vi "GV_YzoomLimit.vi"(6 "Zoom In/Out":bool, 8 "error in (no error)":errorcluster, 11 "Gviewer in":refnum<class "Gviewer.lvclass">) -> (0 "error out":errorcluster, 1 "Allowed":bool, 3 "Gviewer out":refnum<class "Gviewer.lvclass">)   [LabVIEW 2020, in "Sgraph_lib_V1.lvlib" / "Gviewer.lvclass"]
doc: "Determine if Y scrollwheel zoom is still allowed (within limits?)"
uses:
  Gviewer.lvclass
  Gviewer.lvclass/Gviewer.ctl
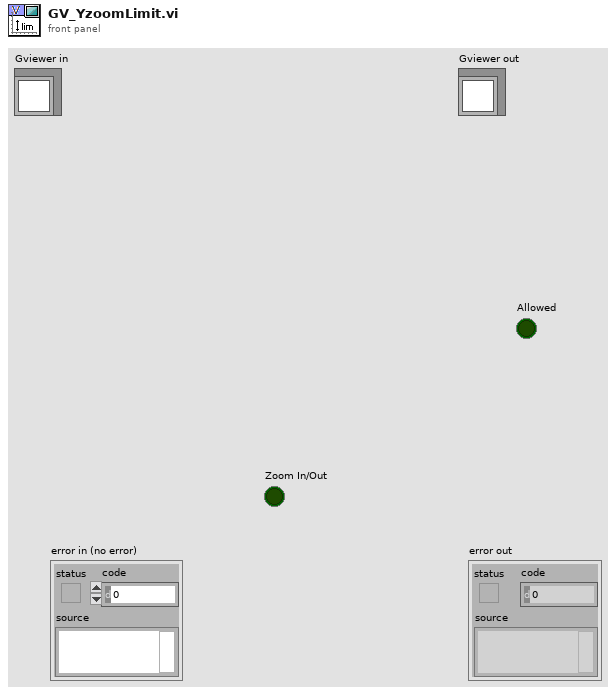
[diagram p1: front panel]
types:
  T1 = typedef "Sgraph_lib_V1.lvlib/Gviewer.lvclass/Typedef_SelProperties.ctl" = cluster{"Color":u32, "LineType":T2, "max":dbl, "min":dbl, "unit":string}
  T2 = typedef "Sgraph_lib_V1.lvlib/Gviewer.lvclass/Typedef_LineType.ctl" = enum16{"num_bare", "num_MinMax_Area", "num_MinMax_Lines", "num_MinMax_Forfor", "num_Max_Area", "num_Max_Line", "num_Max_Forfor", "num_Min_Area", "num_Min_Line", "num_Min_Fosfor", "Boolean_Line_01", "Boolean_Area_01", "Boolean_Fosfor_01", "Boolean_Line_TF", "Boolean_Area_TF", "Boolean_Fosfor_TF", "Boolean_OnOff_Line", "Boolean_OnOff_Area", "Boolean_OnOff_Fosfor", "Boolean_spare", "StringEvent_Line", "StringEvent_TimeLine"}
  T3 = cluster{"data":dbl[], "max":dbl[], "min":dbl[], "Status":u32[]}[]
  T4 = typedef "LVRectTypeDef.ctl" = cluster{"Left":i16, "Top":i16, "Right":i16, "Bottom":i16}
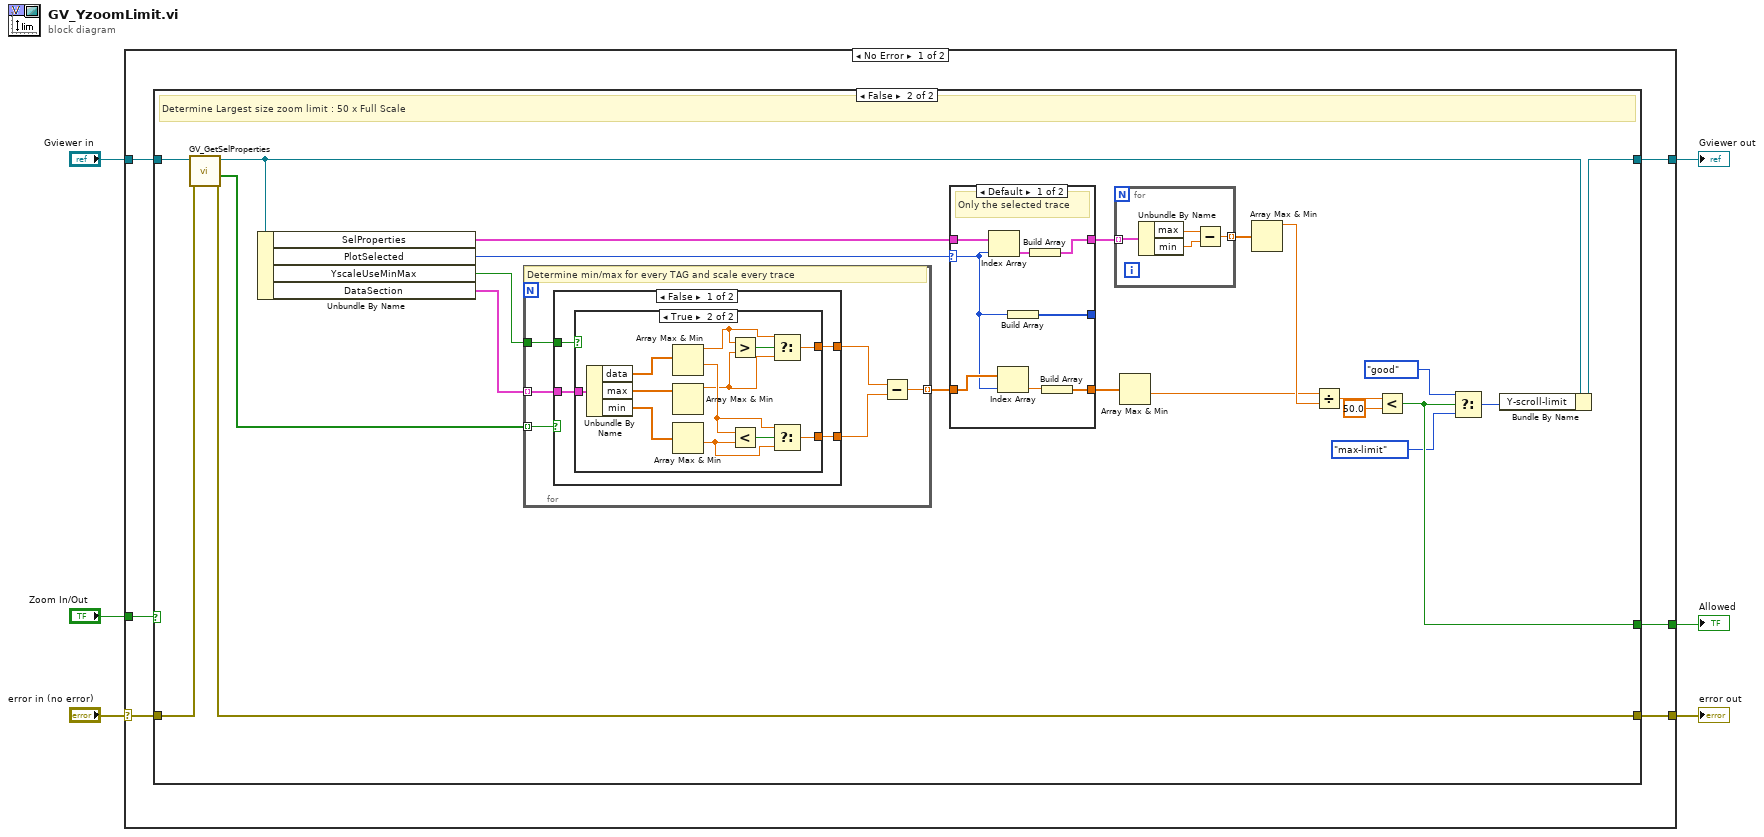
[diagram p0: block diagram]
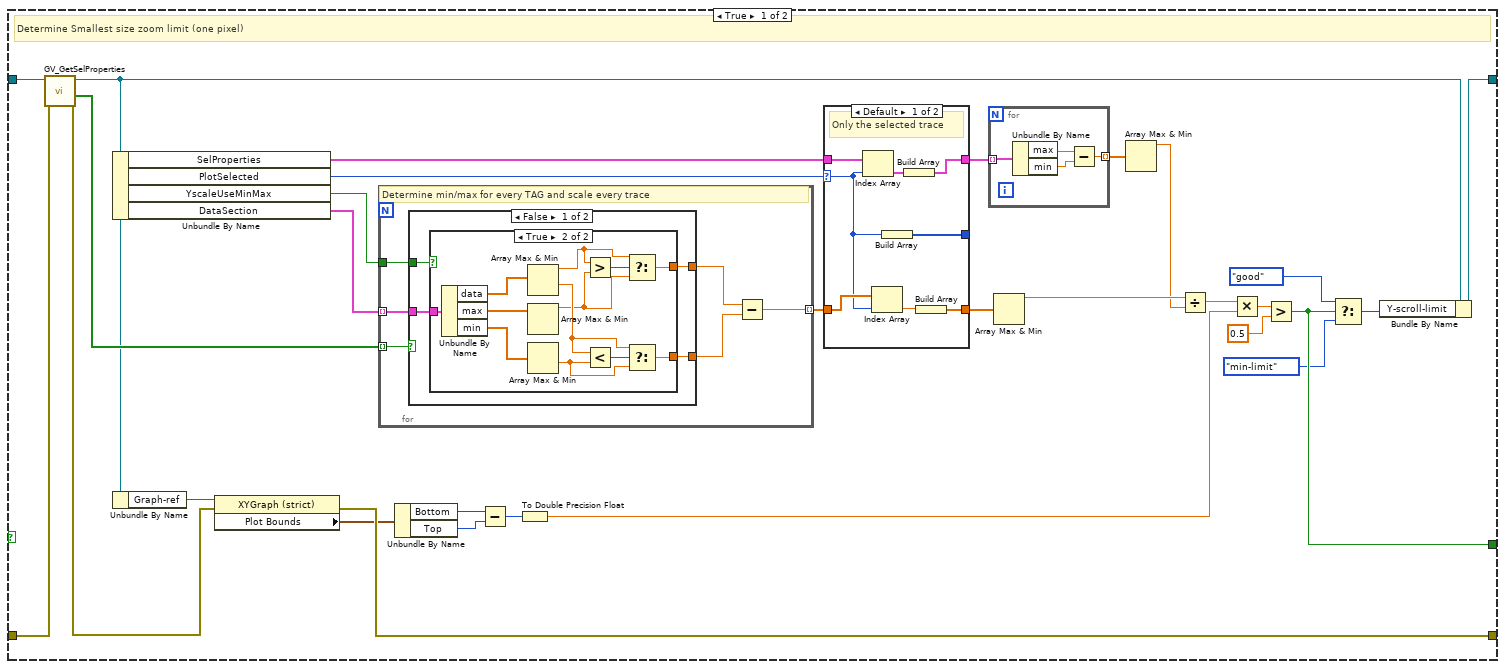
[diagram p2: hidden frame]
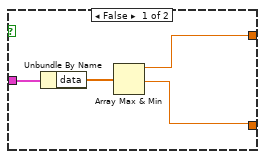
[diagram p3: hidden frame]
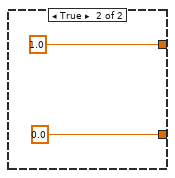
[diagram p4: hidden frame]
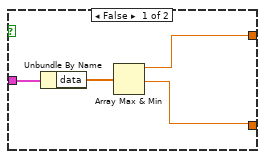
[diagram p6: hidden frame]
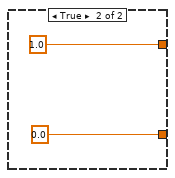
[diagram p7: hidden frame]
diagram:
  n1 = case shown="No Error" "error in (no error)" {
    selector: "error in (no error)" -> [w11 w154]
    tunnel: [w9 w154] -> w5
    tunnel: [w10 w153] -> w3
    tunnel: "Gviewer in" -> [w12 w153]
    tunnel: [w8 _] -> w2
    tunnel: "Zoom In/Out" -> [w7 _]
    frame No Error {
      n2 = case shown="False" w7 {
        tunnel: w12 -> [w40 w106]
        tunnel: w11 -> [w38 w104]
        tunnel: [w15 w87] -> w10
        tunnel: [w31 w97] -> w9
        tunnel: [w17 w92] -> w8
        frame True {
          # "Determine Smallest size zoom limit (one pixel)"
          n3 = call "GV_GetSelProperties.vi"("error in (no error)"=w38, "Gviewer in"=w40) -> ("error out"=w32:errorcluster, "Bool_id"=w39:bool[], "Gviewer out"=w16:refnum<class "Gviewer.lvclass">)  [unwired: 6 in, 1 out]
          n4 = Unbundle By Name(w16) -> ("SelProperties"=w37:T1[], "PlotSelected"=w42:i32, "YscaleUseMinMax"=w41:bool, "DataSection"=w36:T3)
          n5 = Unbundle By Name(w16) -> ("Graph-ref"=w33:refnum<vi>)
          n6 = property class="XYGraph (strict)"(reference=w33, error in=w32) -> (error out=w31:errorcluster, "Plot Bounds"=w30:T4)  [unwired: 1 out]
          n7 = for {
            tunnel: w41 -> [w52]
            tunnel: w36 -> [w51] mode=indexing
            tunnel: w39 -> [w50] mode=indexing
            tunnel: [w47] -> w35 mode=indexing
            # "Determine min/max for every TAG and scale every trace"
            n8 = case shown="False" w50 {
              tunnel: w52 -> [w56 _]
              tunnel: w51 -> [w55 _]
              tunnel: [w54 1.0] -> w49
              tunnel: [w53 0.0] -> w48
              frame False {
                n9 = case shown="True" w56 {
                  tunnel: w55 -> [w59 w72]
                  tunnel: [w58 w64] -> w54
                  tunnel: [w57 w63] -> w53
                  frame False {
                    n10 = Unbundle By Name(w59) -> ("data"=w60:dbl[])
                    n11 = Array Max & Min(array=w60) -> (max value=w58:dbl, min value=w57:dbl)  [unwired: 2 out]
                  }
                  frame True {
                    n12 = Unbundle By Name(w72) -> ("data"=w71:dbl[], "max"=w70:dbl[], "min"=w69:dbl[])
                    n13 = Array Max & Min(array=w71) -> (max value=w62:dbl, min value=w65:dbl)  [unwired: 2 out]
                    n14 = Array Max & Min(array=w70) -> (max value=w61:dbl)  [unwired: 3 out]
                    n15 = Array Max & Min(array=w69) -> (min value=w66:dbl)  [unwired: 3 out]
                    n16 = Greater?(x=w62, y=w61) -> (0:w68:bool)
                    n17 = Less?(x=w65, y=w66) -> (x < y?=w67:bool)
                    n18 = Select(t=w62, s=w68, f=w61) -> (s? t:f=w64:dbl)
                    n19 = Select(t=w65, s=w67, f=w66) -> (s? t:f=w63:dbl)
                  }
                }
              }
              frame True {
              }
            }
            n20 = Subtract(x=w49, y=w48) -> (x-y=w47:dbl)
          }
          n21 = Unbundle By Name(w30) -> ("Bottom"=w29:i16, "Top"=w28:i16)
          n22 = Subtract(x=w29, y=w28) -> (x-y=w24:i16)
          n23 = To Double Precision Float(number=w24) -> (double precision float=w21:dbl)
          n24 = case shown="Default" w42 {
            selector: w42 -> [w77 _]
            tunnel: w37 -> [w81 w83]
            tunnel: [w82 w83] -> w27
            tunnel: [w79 w85] -> _
            tunnel: w35 -> [w78 w84]
            tunnel: [w75 w84] -> w34
            frame Default {
              # "Only the selected trace"
              n25 = Index Array(array=w81, index=w77) -> (element=w80:T1)
              n26 = Index Array(array=w78, index=w77) -> (element=w76:dbl)
              n27 = Build Array(w77) -> (w79:i32[])
              n28 = Build Array(w80) -> (w82:T1[])
              n29 = Build Array(w76) -> (w75:dbl[])
            }
            frame -1 {
              # "All traces"
              n30 = for {
                tunnel: [w86] -> w85 mode=indexing
                tunnel: w83 -> [_] mode=indexing
                i -> [w86]
              }
            }
          }
          n31 = for {
            tunnel: w27 -> [w46] mode=indexing
            tunnel: [w43] -> w26 mode=indexing
            n32 = Unbundle By Name(w46) -> ("max"=w45:dbl, "min"=w44:dbl)
            n33 = Subtract(x=w45, y=w44) -> (x-y=w43:dbl)
          }
          n34 = Array Max & Min(array=w34) -> (max value=w23:dbl)  [unwired: 3 out]
          n35 = Array Max & Min(array=w26) -> (max value=w22:dbl)  [unwired: 3 out]
          n36 = Divide(x=w23, y=w22) -> (x/y=w25:dbl)
          n37 = Multiply(x=w25, y=w21) -> (x*y=w20:dbl)
          n38 = Greater?(x=w20, y=0.5) -> (0:w17:bool)
          n39 = Select(t=enum16{"good", "min-limit", "max-limit"}."good" ("Y-scroll-limit"), s=w17, f=enum16{"good", "min-limit", "max-limit"}."min-limit" ("Y-scroll-limit")) -> (s? t:f=w18:enum16{"good", "min-limit", "max-limit"})
          n40 = Bundle By Name(cluster=w16, "Y-scroll-limit"=w18) -> (w15:refnum<class "Gviewer.lvclass">)
        }
        frame False {
          # "Determine Largest size zoom limit : 50 x Full Scale"
          n41 = call "GV_GetSelProperties.vi"("error in (no error)"=w104, "Gviewer in"=w106) -> ("error out"=w97:errorcluster, "Bool_id"=w105:bool[], "Gviewer out"=w88:refnum<class "Gviewer.lvclass">)  [unwired: 6 in, 1 out]
          n42 = Unbundle By Name(w88) -> ("SelProperties"=w103:T1[], "PlotSelected"=w108:i32, "YscaleUseMinMax"=w107:bool, "DataSection"=w102:T3)
          n43 = for {
            tunnel: w107 -> [w118]
            tunnel: w102 -> [w117] mode=indexing
            tunnel: w105 -> [w116] mode=indexing
            tunnel: [w113] -> w101 mode=indexing
            # "Determine min/max for every TAG and scale every trace"
            n44 = case shown="False" w116 {
              tunnel: w118 -> [w122 _]
              tunnel: w117 -> [w121 _]
              tunnel: [w120 1.0] -> w115
              tunnel: [w119 0.0] -> w114
              frame False {
                n45 = case shown="True" w122 {
                  tunnel: w121 -> [w125 w138]
                  tunnel: [w124 w130] -> w120
                  tunnel: [w123 w129] -> w119
                  frame False {
                    n46 = Unbundle By Name(w125) -> ("data"=w126:dbl[])
                    n47 = Array Max & Min(array=w126) -> (max value=w124:dbl, min value=w123:dbl)  [unwired: 2 out]
                  }
                  frame True {
                    n48 = Unbundle By Name(w138) -> ("data"=w137:dbl[], "max"=w136:dbl[], "min"=w135:dbl[])
                    n49 = Array Max & Min(array=w137) -> (max value=w128:dbl, min value=w131:dbl)  [unwired: 2 out]
                    n50 = Array Max & Min(array=w136) -> (max value=w127:dbl)  [unwired: 3 out]
                    n51 = Array Max & Min(array=w135) -> (min value=w132:dbl)  [unwired: 3 out]
                    n52 = Greater?(x=w128, y=w127) -> (0:w134:bool)
                    n53 = Less?(x=w131, y=w132) -> (x < y?=w133:bool)
                    n54 = Select(t=w128, s=w134, f=w127) -> (s? t:f=w130:dbl)
                    n55 = Select(t=w131, s=w133, f=w132) -> (s? t:f=w129:dbl)
                  }
                }
              }
              frame True {
              }
            }
            n56 = Subtract(x=w115, y=w114) -> (x-y=w113:dbl)
          }
          n57 = case shown="Default" w108 {
            selector: w108 -> [w143 _]
            tunnel: w103 -> [w147 w149]
            tunnel: [w148 w149] -> w99
            tunnel: [w145 w151] -> _
            tunnel: w101 -> [w144 w150]
            tunnel: [w141 w150] -> w100
            frame Default {
              # "Only the selected trace"
              n58 = Index Array(array=w147, index=w143) -> (element=w146:T1)
              n59 = Index Array(array=w144, index=w143) -> (element=w142:dbl)
              n60 = Build Array(w143) -> (w145:i32[])
              n61 = Build Array(w146) -> (w148:T1[])
              n62 = Build Array(w142) -> (w141:dbl[])
            }
            frame -1 {
              # "All traces"
              n63 = for {
                tunnel: [w152] -> w151 mode=indexing
                tunnel: w149 -> [_] mode=indexing
                i -> [w152]
              }
            }
          }
          n64 = for {
            tunnel: w99 -> [w112] mode=indexing
            tunnel: [w109] -> w98 mode=indexing
            n65 = Unbundle By Name(w112) -> ("max"=w111:dbl, "min"=w110:dbl)
            n66 = Subtract(x=w111, y=w110) -> (x-y=w109:dbl)
          }
          n67 = Array Max & Min(array=w100) -> (min value=w93:dbl)  [unwired: 3 out]
          n68 = Array Max & Min(array=w98) -> (max value=w94:dbl)  [unwired: 3 out]
          n69 = Divide(x=w93, y=w94) -> (x/y=w96:dbl)
          n70 = Less?(x=w96, y=50.0) -> (x < y?=w92:bool)
          n71 = Select(t=enum16{"good", "min-limit", "max-limit"}."good" ("Y-scroll-limit"), s=w92, f=enum16{"good", "min-limit", "max-limit"}."max-limit" ("Y-scroll-limit")) -> (s? t:f=w89:enum16{"good", "min-limit", "max-limit"})
          n72 = Bundle By Name(cluster=w88, "Y-scroll-limit"=w89) -> (w87:refnum<class "Gviewer.lvclass">)
        }
      }
    }
    frame Error {
    }
  }
  "error out" <- w5
  "Gviewer out" <- w3
  "Allowed" <- w2
